vi "IRCalibration.vi"(10 "Stop Point":dbl=9.0 format="%#_13g", 11 "Duty Cycle (-100 to + 100)":dbl=10.0 format="%#_13g") -> (2 "Boolean":bool, 3 "interpolation value":dbl)   [LabVIEW 2017]
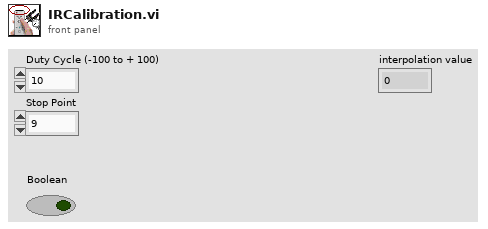
[diagram p1: front panel]
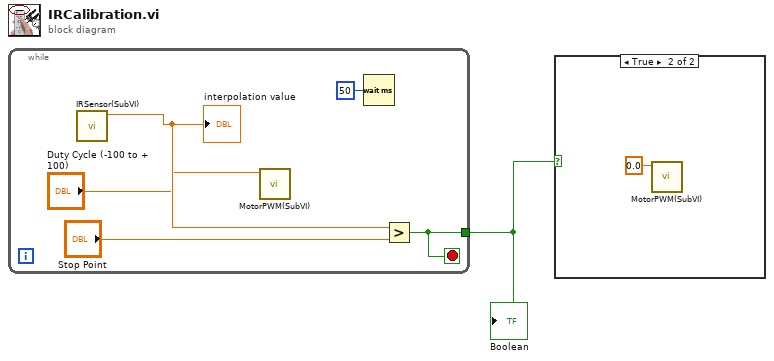
[diagram p0: block diagram]
diagram:
  n1 = while {
    tunnel: [w4] -> w1
    stop <- w4 stop-if-true
    n2 = call "IRSensor(SubVI).vi"() -> ("interpolation value"=w5:dbl)  [unwired: 11 in]
    "interpolation value" <- w5
    n3 = call "MotorPWM(SubVI).vi"("Duty Cycle (-100 to + 100)"="Duty Cycle (-100 to + 100)") -> ()  [unwired: 11 in]
    n4 = Wait (ms)(milliseconds to wait=u32 50) -> ()  [unwired: 1 out]
    n5 = Greater?(x=w5, y="Stop Point") -> (0:w4:bool)
  }
  "Boolean" <- w1
  n6 = case shown="True" w1 {
    frame False {
    }
    frame True {
      n7 = call "MotorPWM(SubVI).vi"("Duty Cycle (-100 to + 100)"=0.0) -> ()  [unwired: 11 in]
    }
  }
